vi "DSF.Engine.BuilderManager.Send Command to Builder.vi"(8 "error in (no error)":errorcluster, 10 "command":T3, 11 "Builder Manager in":refnum<class "DSF.Engine.BuilderManager.lvclass">) -> (0 "error out":errorcluster, 1 "expected response":T1, 2 "Builder":refnum<class "DSF.Engine.Builder.lvclass">, 3 "Builder Manager out":refnum<class "DSF.Engine.BuilderManager.lvclass">)   [LabVIEW 2017, in "DSF.Engine.lvlib" / "DSF.Engine.BuilderManager.lvclass"]
uses:
  DSF.Engine.BuilderManager.lvclass
  Interface/DSF.Engine.Interface.Builder.Command Data.ctl
  Interface/DSF.Engine.Interface.Builder.Command.ctl
  Builder/DSF.Engine.Builder.lvclass
  Interface/DSF.Engine.Interface.Builder.Response Data.ctl
  Interface/DSF.Engine.Interface.Builder.Response.ctl
  Builder/DSF.Engine.Builder.lvclass/DSF.Engine.Builder.ctl
  Interface/DSF.Engine.Interface.Builder.Write.Command.vi
  Interface/DSF.Engine.Interface.Builder.lvclass
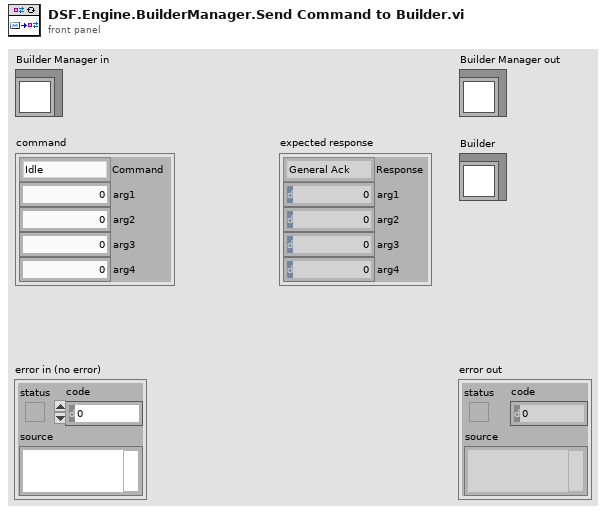
[diagram p1: front panel]
types:
  T1 = typedef "DSF.Engine.lvlib/DSF.Engine.Interface.Builder.lvclass/DSF.Engine.Interface.Builder.Response Data.ctl" = cluster{"Response":T2, "arg1":i32, "arg2":i32, "arg3":i32, "arg4":i32}
  T2 = typedef "DSF.Engine.lvlib/DSF.Engine.Interface.Builder.lvclass/DSF.Engine.Interface.Builder.Response.ctl" = enum8{"General Ack", "Initialize Complete", "Build Complete", "Parse Complete", "Shutdown Ack"}
  T3 = typedef "DSF.Engine.lvlib/DSF.Engine.Interface.Builder.lvclass/DSF.Engine.Interface.Builder.Command Data.ctl" = cluster{"Command":T4, "arg1":i32, "arg2":i32, "arg3":i32, "arg4":i32}
  T4 = typedef "DSF.Engine.lvlib/DSF.Engine.Interface.Builder.lvclass/DSF.Engine.Interface.Builder.Command.ctl" = enum8{"Idle", "Initialize", "Build Buffer", "Parse Buffer", "Shutdown"}
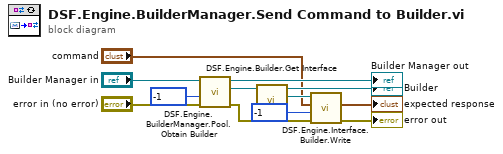
[diagram p0: block diagram]
diagram:
  n1 = call "DSF.Engine.BuilderManager.Pool.Obtain Builder.vi"("error in (no error)"="error in (no error)", "timeout in ms (250)"=-1, "Builder Manager in"="Builder Manager in") -> ("error out"=w11:errorcluster, "Builder"=w12:refnum<class "DSF.Engine.Builder.lvclass">, "Builder Manager out"=→"Builder Manager out":refnum<class "DSF.Engine.BuilderManager.lvclass">)  [unwired: 6 in]
  n2 = call "DSF.Engine.Builder.Get Interface.vi"("Builder in"=w12) -> ("Builder Interface"=w3:refnum<class "DSF.Engine.Interface.Builder.lvclass">, "Builder out"=→"Builder":refnum<class "DSF.Engine.Builder.lvclass">)  [unwired: 9 in]
  n3 = call-poly "DSF.Engine.Interface.Builder.Write.vi"("error in (no error)"=w11, "timeout in ms (0)"=-1, "command"="command", "Builder Interface in"=w3) -> ("error out"=→"error out":errorcluster, "expected response"=→"expected response":T1)  [unwired: 4 in, 2 out]
